vi "DynamixelConfigureAngleLimits.vi"(0 "VISA resource name":refnum<visa-resource-name>, 5 "Motor ID (0)":u8, 7 "Clockwise Angle Limit (0 deg)":dbl, 9 "Counter-Clockwise Angle Limit (300 deg)":dbl=300.0, 11 "error in (no error)":errorcluster) -> (4 "VISA resource name out":refnum<visa-resource-name>, 15 "error out":errorcluster)   [LabVIEW 2013]
doc: "Changes the ID of a motor."
uses:
  <instrlib>/Dynamixel Motor/Dynamixel Motor.lvlib
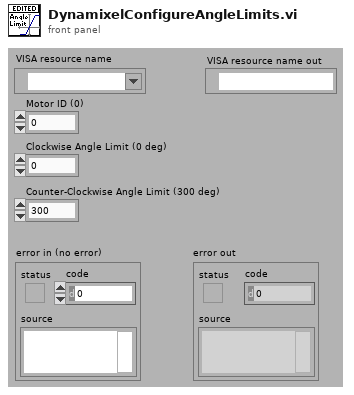
[diagram p1: front panel]
types:
  T1 = enum16{"big-endian, network order", "native, host order", "little-endian"}
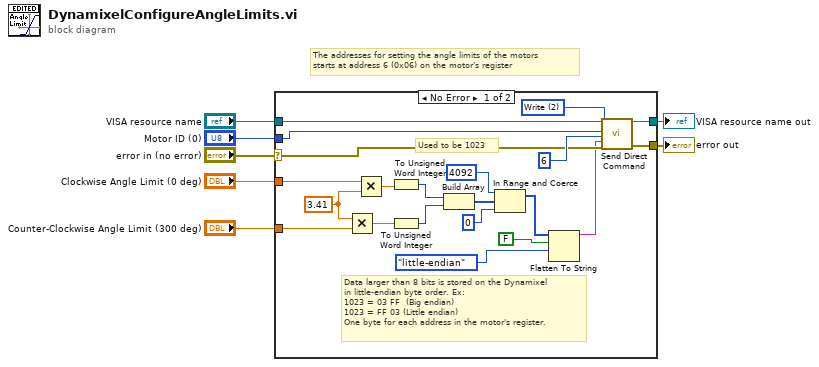
[diagram p0: block diagram]
diagram:
  # "The addresses for setting the angle limits of the motors\nstarts at address 6 (0x06) on the motor's register"
  n1 = case shown="No Error" "error in (no error)" {
    selector: "error in (no error)" -> [w19 w30]
    tunnel: [w22 w30] -> w6
    tunnel: "VISA resource name" -> [w25 w29]
    tunnel: [w23 w29] -> w4
    tunnel: "Motor ID (0)" -> [w21 _]
    tunnel: "Clockwise Angle Limit (0 deg)" -> [w27 _]
    tunnel: "Counter-Clockwise Angle Limit (300 deg)" -> [w26 _]
    frame No Error {
      w24 = u16 2 items=["Ping", "Read", "Write", "Registered Write", "Action", "Reset", "Sync Write"] ("Select Action")
      w28 = 3.41
      # "Used to be 1023"
      # "Data larger than 8 bits is stored on the Dynamixel \nin little-endian byte order. Ex:\n1023 = 03 FF  (Big endian)\n1023 = FF 03 (Little endian)\nOne byte for each address in the motor's register."
      n2 = Multiply(x=w28, y=w26) -> (x*y=w15:dbl)
      n3 = Multiply(x=w27, y=w28) -> (x*y=w16:dbl)
      n4 = To Unsigned Word Integer(number=w16) -> (unsigned 16bit integer=w14:u16)
      n5 = To Unsigned Word Integer(number=w15) -> (unsigned 16bit integer=w13:u16)
      n6 = Build Array(w14, w13) -> (w12:u16[])
      n7 = In Range and Coerce(upper limit=u16 4092, x=w12, lower limit=u16 0) -> (coerced(x)=w10:u16[])  [unwired: 1 out]
      n8 = Flatten To String(anything=w10, prepend array or string size? (T)=FALSE, byte order (0:big-endian, network order)=T1."little-endian") -> (data string=w11:string)  [unwired: 1 in, 2 out]
      n9 = call <instrlib>:"Send Direct Command.vi"("VISA resource name"=w25, "Select Action"=w24, "Motor ID (0)"=w21, "Address"=u8 6, "Parameters"=w11, "Error in (no error)"=w19) -> ("VISA resource name out"=w23:refnum<visa-resource-name>, "Error out"=w22:errorcluster)  [unwired: 11 in, 1 out]
    }
    frame Error {
    }
  }
  "VISA resource name out" <- w4
  "error out" <- w6
